vi "Channels Page.vi"(8 "error in (no error)":errorcluster, 11 "Node Ptr":T1 format="%.0x") -> (0 "error out":errorcluster)   [LabVIEW 2019, in "Telemetry System Explorer.lvlib"]
uses:
  Telemetry System Explorer.lvlib
  <vilib>/NI VeriStand/Custom Device API/Custom Device Item Ref.ctl
  <vilib>/NI VeriStand/Custom Device API/Get Item Property (Boolean).vi
  <vilib>/NI VeriStand/Custom Device API/Custom Device API.lvlib
panel:
  in  "Remove":bool
  in  "Logged Channels":i32[](listbox)
  in  "SHDocVw.IWebBrowser":refnum<k7>(container)
  in  "General Header":cluster{"Section Name":string}={"Section Name"="General Page Settings"}
  in  "Description":string
  in  "Name":string
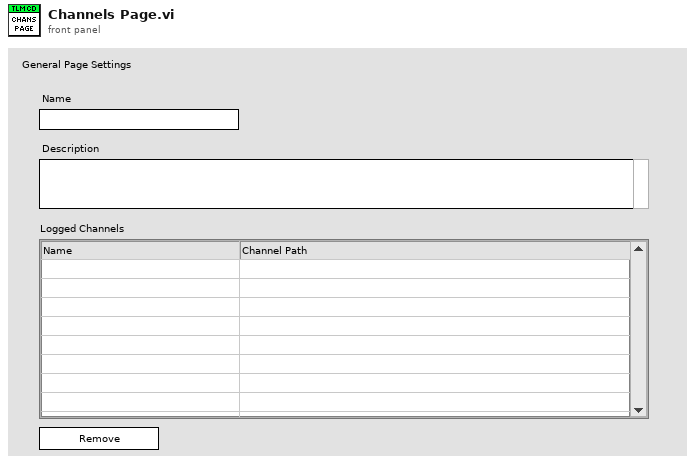
[diagram p1: front panel]
types:
  T1 = typedef "Custom Device API.lvlib/Custom Device Item Ref.ctl" = u64
  T2 = typedef "Custom Device API.lvlib/Custom Device Item Info.ctl" = cluster{"Name":string, "Is Channel":bool, "GUID":string, "Is Waveform":bool}
  T3 = typedef "Custom Device API.lvlib/Custom Device Commands.ctl" = enum16{"Default", "Item renamed", "Shutdown", "Dynamic button pressed"}
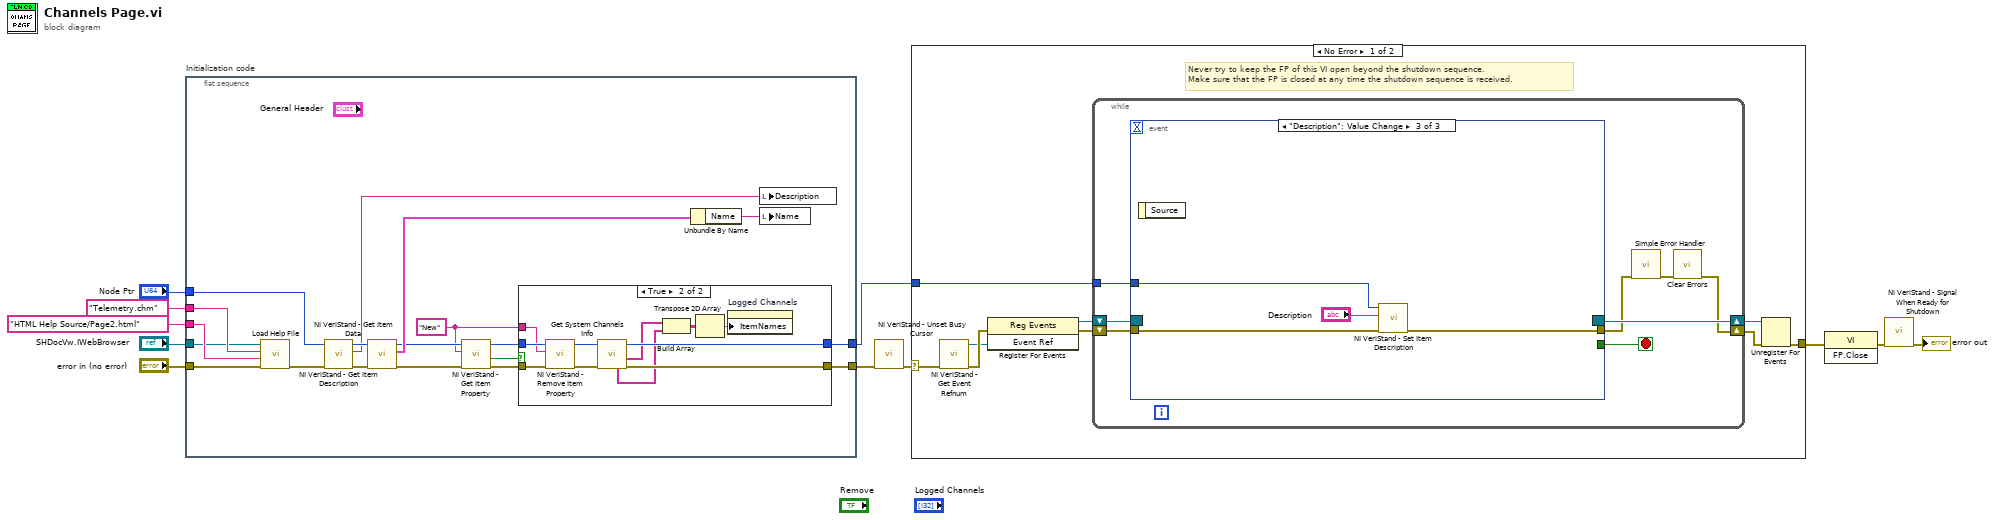
[diagram p0: block diagram]
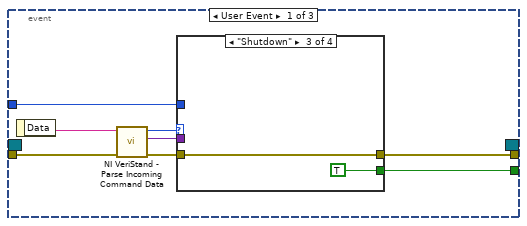
[diagram p3: hidden frame]
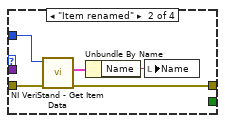
[diagram p5: hidden frame]
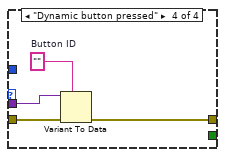
[diagram p6: hidden frame]
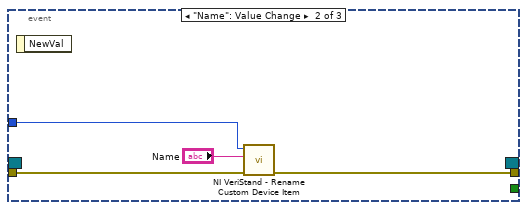
[diagram p7: hidden frame]
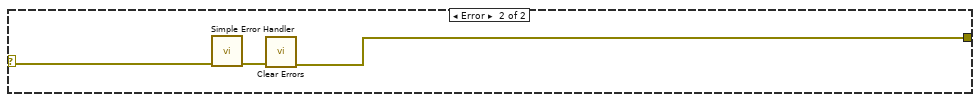
[diagram p8: hidden frame]
diagram:
  n1 = flat-sequence "Initialization code" {
    tunnel: "error in (no error)" -> [w24]
    tunnel: "Node Ptr" -> [w27]
    tunnel: [w15] -> w7
    tunnel: [w13] -> w4
    tunnel: "SHDocVw.IWebBrowser" -> [w20]
    tunnel: "HTML Help Source/Page2.html" ("CD_CHM_Section") -> [w22]
    tunnel: "Telemetry.chm" ("CD_CHM_FileName") -> [w21]
    frame #0 {
      w12 = "New" ("Property Name")
      n2 = call "Load Help File.vi"("error in (no error)"=w24, "HTML File to Load"=w22, "Main CHM File"=w21, "Browser"=w20) -> ("error out"=w23:errorcluster)  [unwired: 7 in]
      n3 = call <vilib>:"NI VeriStand - Get Item Description.vi"("error in (no error)"=w23, "Item Ref in"=w27) -> ("error out"=w29:errorcluster, "Description"=w25:string, "Item Ref out"=w30:T1)  [unwired: 7 out]
      n4 = call <vilib>:"NI VeriStand - Get Item Data.vi"("error in (no error)"=w29, "Item Ref in"=w30) -> ("error out"=w19:errorcluster, "Item Info"=w28:T2, "Item Ref out"=w18:T1)  [unwired: 7 out]
      n5 = call-poly <vilib>:"NI VeriStand - Get Item Property.vi"("error in (no error)"=w19, "Property Name"=w12, "Item Ref in"=w18) -> ("error out"=w16:errorcluster, "Value"=w17:bool, "Item Ref out"=w14:T1)  [unwired: 5 in, 1 out]
      n6 = case shown="True" w17 {
        tunnel: w16 -> [w31 w43]
        tunnel: [w31 w37] -> w15
        tunnel: w14 -> [w32 w42]
        tunnel: [w32 w39] -> w13
        tunnel: w12 -> [_ w41]
        frame False {
        }
        frame True {
          n7 = call <vilib>:"NI VeriStand - Remove Item Property.vi"("error in (no error)"=w43, "Property Name"=w41, "Item Ref in"=w42) -> ("error out"=w38:errorcluster, "Item Ref out"=w40:T1)  [unwired: 6 in, 1 out]
          n8 = call "Get System Channels Info.vi"("error in (no error)"=w38, "Item Ref in"=w40) -> ("error out"=w37:errorcluster, "Channel Names"=w36:string[], "Item Ref out"=w39:T1, "Channel Paths"=w35:string[])  [unwired: 5 in, 1 out]
          n9 = Build Array(w36, w35) -> (w34:string[][])
          n10 = Transpose 2D Array(2D array=w34) -> (transposed array=w33:string[][])
          n11 = property on="Logged Channels" class="MCListbox (strict)"("ItemNames"=w33) -> ()  [unwired: 2 in, 2 out]
        }
      }
      n12 = Unbundle By Name(w28) -> ("Name"=w26:string)
      n13 = local write "Description"(w25) -> ()
      n14 = local write "Name"(w26) -> ()
    }
  }
  n15 = call <vilib>:"NI VeriStand - Unset Busy Cursor.vi"("error in (no error)"=w7) -> ("error out"=w6:errorcluster)  [unwired: 10 out]
  n16 = case shown="No Error" w6 {
    selector: w6 -> [w44 w91]
    tunnel: [w49 w89] -> w11
    tunnel: w4 -> [w45 _]
    frame No Error {
      # "Never try to keep the FP of this VI open beyond the shutdown sequence.\nMake sure that the FP is closed at any time the shutdown sequence is received."
      n17 = call <vilib>:"NI VeriStand - Get Event Refnum.vi"("error in (no error)"=w44) -> ("error out"=w52:errorcluster, "Event Ref"=w48:refnum<user-event>)  [unwired: 9 out]
      n18 = register-events(error in=w52, w48) -> (reference out=w46:refnum<event-registration>, error out=w47:errorcluster)  [unwired: 1 in]
      n19 = while {
        tunnel: w45 -> [w56]
        shift-right: [w53] -> w50
        shift-left: w47 -> [w59]
        shift-right: [w60] -> w51
        shift-left: w46 -> [w58]
        stop <- w57 stop-if-true
        n20 = event shown="[2] \"Description\": Value Change" {
          selector: w58 -> [_ _ _]
          dyn-events: [_ _ _] -> w60
          timeout: _ -> [_ _ _]
          tunnel: w59 -> [w68 w84 w87]
          tunnel: [w64 _ _] -> w57
          tunnel: [w63 w83 w86] -> w55
          tunnel: w56 -> [w62 w82 w88]
          event User Event {
            n21 = event-data() -> ("Data"=w67:string)  [unwired: 1 out]
            n22 = call <vilib>:"NI VeriStand - Parse Incoming Command Data.vi"("error in (no error)"=w68, "Incoming data"=w67) -> ("error out"=w66:errorcluster, "Outgoing data"=w61:variant, "Action"=w65:T3)  [unwired: 7 out]
            n23 = case shown="\"Shutdown\"" w65 {
              tunnel: w66 -> [w69 w74 w75 w80]
              tunnel: [_ _ TRUE _] -> w64
              tunnel: [w69 w71 w75 w77] -> w63
              tunnel: w62 -> [_ w73 _ _]
              tunnel: w61 -> [_ _ _ w79]
              frame "Default", Default {
              }
              frame "Item renamed" {
                n24 = call <vilib>:"NI VeriStand - Get Item Data.vi"("error in (no error)"=w74, "Item Ref in"=w73) -> ("error out"=w71:errorcluster, "Item Info"=w72:T2)  [unwired: 8 out]
                n25 = Unbundle By Name(w72) -> ("Name"=w70:string)
                n26 = local write "Name"(w70) -> ()
              }
              frame "Shutdown" {
              }
              frame "Dynamic button pressed" {
                w78 = ""  # Button ID
                n27 = Variant To Data(error in=w80, type=w78, Variant=w79) -> (error out=w77:errorcluster)  [unwired: 1 out]
              }
            }
          }
          event "Name": Value Change {
            n28 = event-data() -> ()  [unwired: 2 out]
            n29 = call <vilib>:"NI VeriStand - Rename Custom Device Item.vi"("error in (no error)"=w84, "New Name"="Name", "Item Ref in"=w82) -> ("error out"=w83:errorcluster)  [unwired: 1 in, 7 out]
          }
          event "Description": Value Change {
            n30 = event-data() -> ()  [unwired: 2 out]
            n31 = call <vilib>:"NI VeriStand - Set Item Description.vi"("error in (no error)"=w87, "Description"="Description", "Item Ref in"=w88) -> ("error out"=w86:errorcluster)  [unwired: 8 out]
          }
        }
        n32 = call <vilib>:"Simple Error Handler.vi"("error in (no error)"=w55) -> ("error out"=w54:errorcluster)  [unwired: 1 in, 7 out]
        n33 = call <vilib>:"Clear Errors.vi"("error in (no error)"=w54) -> ("error out"=w53:errorcluster)  [unwired: 1 in, 5 out]
      }
      n34 = Unregister For Events(event registration refnum=w51, error in=w50) -> (error out=w49:errorcluster)
    }
    frame Error {
      n35 = call <vilib>:"Simple Error Handler.vi"("error in (no error)"=w91) -> ("error out"=w90:errorcluster)  [unwired: 1 in, 7 out]
      n36 = call <vilib>:"Clear Errors.vi"("error in (no error)"=w90) -> ("error out"=w89:errorcluster)  [unwired: 1 in, 5 out]
    }
  }
  n37 = invoke class="VI" method="FP.Close"(error in=w11) -> (error out=w10:errorcluster)  [unwired: 2 in, 2 out]
  n38 = call <vilib>:"NI VeriStand - Signal When Ready for Shutdown.vi"("error in (no error)"=w10) -> ("error out"=→"error out":errorcluster)  [unwired: 10 out]
